vi "SUB_KILL_TFTPD32_TASK.vi"() -> ()   [LabVIEW 2011]
panel:
  out "code":i32
  out "standard output":string
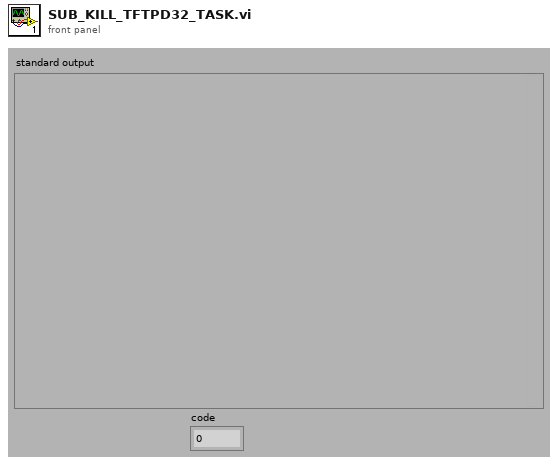
[diagram p1: front panel]
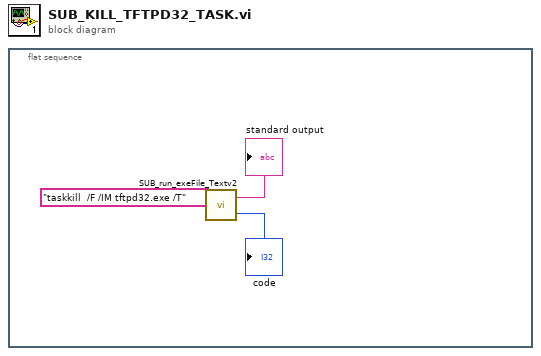
[diagram p0: block diagram]
diagram:
  n1 = flat-sequence {
    frame #0 {
      n2 = call "SUB_run_exeFile_Textv2.vi"("exe filename"="taskkill  /F /IM tftpd32.exe /T") -> ("code"=→"code":i32, "standard output"=→"standard output":string)  [unwired: 1 in]
    }
  }
